vi "LoadParametersFromFile.vi"(8 "error in (no error)":errorcluster, 10 "Config file path":path, 11 "CDependencyInspection in":refnum<class "CDependencyInspection.lvclass">) -> (0 "error out":errorcluster, 3 "CDependencyInspection out":refnum<class "CDependencyInspection.lvclass">)   [LabVIEW 2020, in "DependencyInspection.lvlib" / "CDependencyInspection.lvclass"]
uses:
  CDependencyInspection.lvclass
  d2aa5e02-a701-478b-bdd8-a180941180cd.vi
  CommonHelpers/CommonHelpers.lvlib
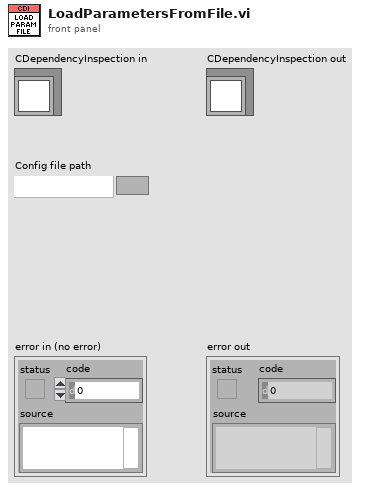
[diagram p1: front panel]
types:
  T1 = cluster{"Config file path":path, "trimmed string":string}
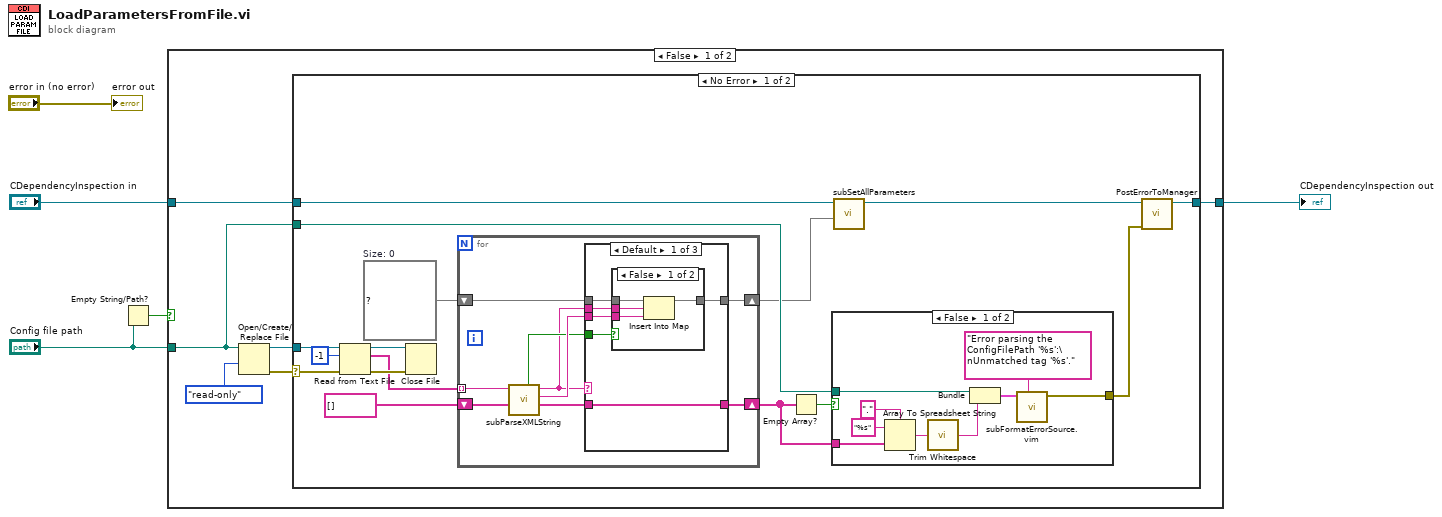
[diagram p0: block diagram]
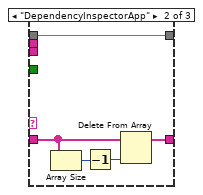
[diagram p3: hidden frame]
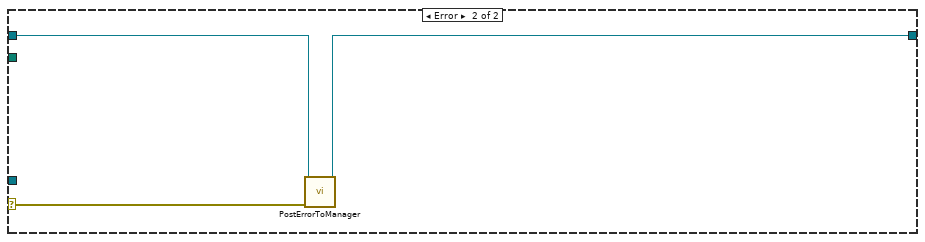
[diagram p6: hidden frame]
diagram:
  n1 = Empty String/Path?(string/path="Config file path") -> (empty?=w5:bool)
  n2 = case shown="False" w5 {
    tunnel: "Config file path" -> [w6 _]
    tunnel: "CDependencyInspection in" -> [w8 w67]
    tunnel: [w7 w67] -> w2
    frame False {
      n3 = Open/Create/Replace File(file path (use dialog)=w6, access (0:read/write)=enum16{"read/write", "read-only", "write-only"}."read-only") -> (refnum out=w10:refnum<file>, error out=w9:errorcluster)  [unwired: 4 in, 1 out]
      n4 = case shown="No Error" w9 {
        selector: w9 -> [w24 w64]
        tunnel: w10 -> [w27 _]
        tunnel: w8 -> [w14 w65]
        tunnel: [w16 w66] -> w7
        tunnel: w6 -> [w20 _]
        frame No Error {
          w15 = map{string, string} {}  # Size: 0
          n5 = Read from Text File(file (use dialog)=w27, count=-1, error in=w24) -> (refnum out=w26:refnum<file>, text=w18:string[], error out=w25:errorcluster)  [unwired: 1 in, 1 out]
          n6 = Close File(refnum=w26, error in=w25) -> ()  [unwired: 2 out]
          n7 = for {
            shift-right: [w35] -> w12
            shift-left: w15 -> [w36]
            tunnel: w18 -> [w34] mode=indexing
            shift-right: [w28] -> w21
            shift-left: string[] [] ("Command line args") -> [w33]
            n8 = call "subParseXMLString.vi"("Parents in"=w33, "input string"=w34) -> ("Parents"=w29:string[], "Value"=w32:string, "Parameter"=w30:string, "Parent?"=w31:bool)  [unwired: 6 in]
            n9 = case shown="Default" w30 {
              tunnel: w36 -> [w42 w52 w54]
              tunnel: [w41 w52 w54] -> w35
              tunnel: w30 -> [w40 _ _]
              tunnel: w32 -> [w39 _ _]
              tunnel: w31 -> [w38 _ _]
              tunnel: w29 -> [w37 w49 w53]
              tunnel: [w37 w48 w53] -> w28
              frame Default {
                n10 = case shown="False" w38 {
                  tunnel: w42 -> [w46 w47]
                  tunnel: [w45 w47] -> w41
                  tunnel: w40 -> [w44 _]
                  tunnel: w39 -> [w43 _]
                  frame False {
                    n11 = Insert Into Map(map in=w46, key=w44, value=w43) -> (map out=w45:map{string, string})  [unwired: 2 out]
                  }
                  frame True {
                  }
                }
              }
              frame "DependencyInspectorApp" {
                n12 = Array Size(array=w49) -> (size(s)=w51:i32)
                n13 = Decrement(x=w51) -> (x-1=w50:i32)
                n14 = Delete From Array(array=w49, index=w50) -> (array with subset deleted=w48:string[])  [unwired: 1 in, 1 out]
              }
              frame "" {
              }
            }
          }
          n15 = Empty Array?(array=w21) -> (empty?=w22:bool)
          n16 = case shown="False" w22 {
            tunnel: w21 -> [w61 _]
            tunnel: [w56 _] -> w17
            tunnel: w20 -> [w60 _]
            frame False {
              n17 = Array To Spreadsheet String(delimiter (Tab)=".", array=w61, 3:"%s" ("format string")) -> (spreadsheet string=w59:string)
              n18 = call <vilib>:"Trim Whitespace.vi"("string"=w59) -> ("trimmed string"=w55:string)  [unwired: 1 in]
              n19 = Bundle("Config file path"=w60, "trimmed string"=w55) -> (w58:T1)  [unwired: 1 in]
              n20 = call "subFormatErrorSource.vim"("format string"="Error parsing the ConfigFilePath '%s':\nUnmatched tag '%s'.", "Parameter cluster"=w58) -> ("Error out"=w56:errorcluster)  [unwired: 9 in]
            }
            frame True {
            }
          }
          n21 = call "subSetAllParameters.vi"("Parameters"=w12, "CDependencyInspection in"=w14) -> ("CDependencyInspection out"=w13:refnum<class "CDependencyInspection.lvclass">)  [unwired: 7 in, 2 out]
          n22 = call-dynamic "PostErrorToManager.vi"("error in (no error)"=w17, "CDependencyInspection in"=w13) -> ("CDependencyInspection out"=w16:refnum<class "CDependencyInspection.lvclass">)  [unwired: 8 in, 1 out]
        }
        frame Error {
          n23 = call-dynamic "PostErrorToManager.vi"("error in (no error)"=w64, "CDependencyInspection in"=w65) -> ("CDependencyInspection out"=w66:refnum<class "CDependencyInspection.lvclass">)  [unwired: 8 in, 1 out]
        }
      }
    }
    frame True {
    }
  }
  "CDependencyInspection out" <- w2
  "error out" <- "error in (no error)"
